vi "Field sweep Generator.vi"(5 "Ramp type":string(combo)="Around origin", 7 "Ramp up first T":bool, 9 "Field Radius":dbl=0.002 format="%#_13g", 10 "Field step":dbl=0.002 format="%#_13g", 11 "Field Origin":dbl=0.002 format="%#_13g") -> (3 "output array":dbl[](array[numeric]))   [LabVIEW 2021]
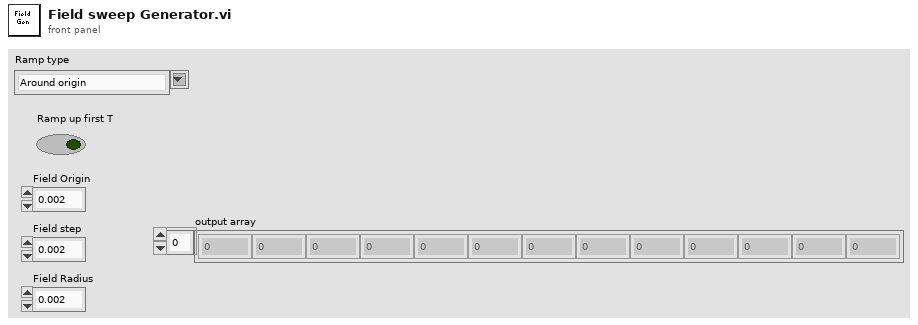
[diagram p1: front panel]
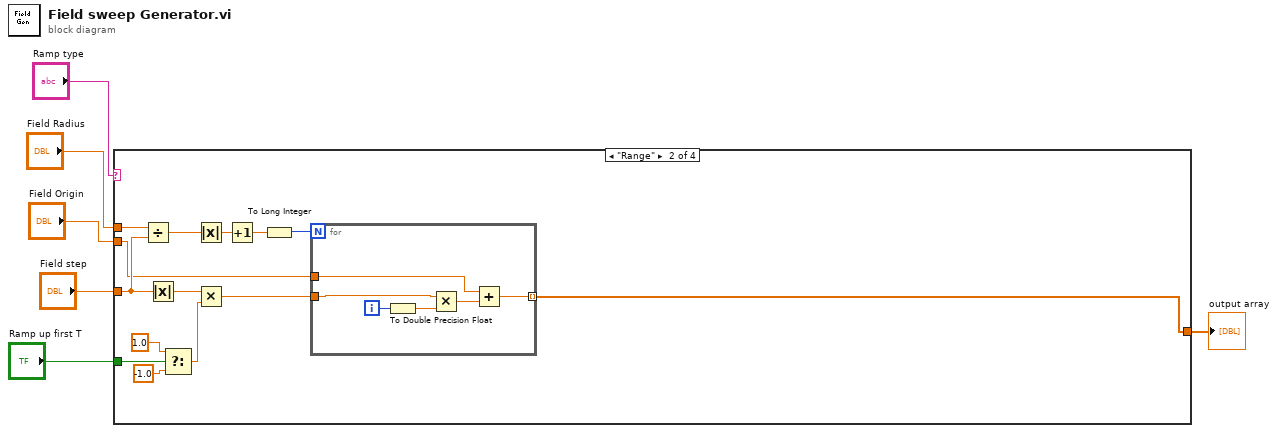
[diagram p0: block diagram]
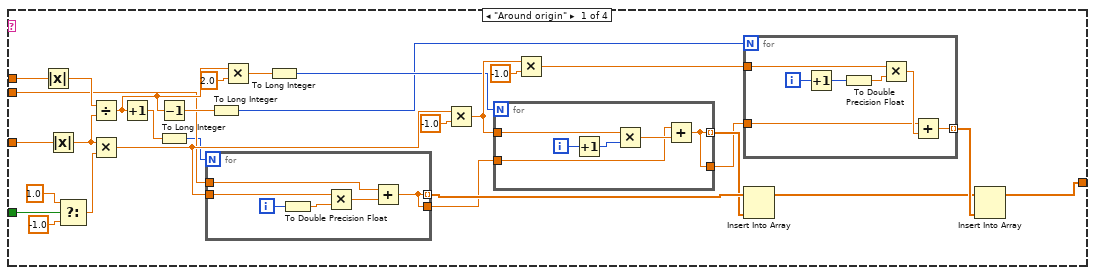
[diagram p2: hidden frame]
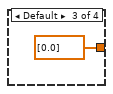
[diagram p3: hidden frame]
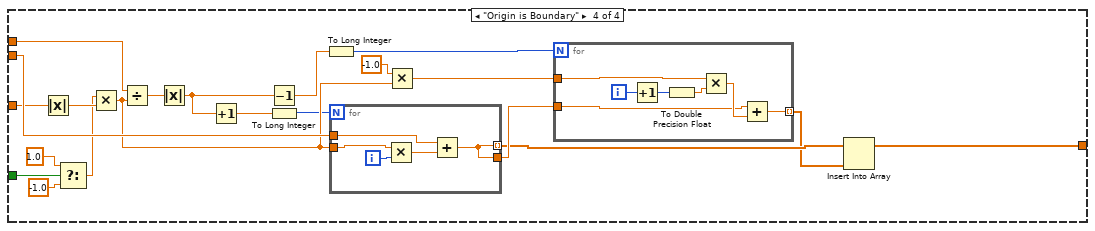
[diagram p4: hidden frame]
diagram:
  n1 = case shown="\"Range\"" "Ramp type" {
    tunnel: [w35 w62 dbl[] [0.0] w84] -> w6
    tunnel: "Ramp up first T" -> [w34 w59 _ w82]
    tunnel: "Field Radius" -> [w31 w68 _ w96]
    tunnel: "Field step" -> [w25 w64 _ w90]
    tunnel: "Field Origin" -> [w10 w63 _ w93]
    frame "Around origin" {
      n2 = Absolute Value(x=w31) -> (abs(x)=w30:dbl)
      n3 = Absolute Value(x=w25) -> (abs(x)=w13:dbl)
      n4 = Select(t=1.0, s=w34, f=-1.0) -> (s? t:f=w11:dbl)
      n5 = Divide(x=w30, y=w13) -> (x/y=w18:dbl)
      n6 = Multiply(x=w13, y=w11) -> (x*y=w12:dbl)
      n7 = Increment(x=w18) -> (x+1=w15:dbl)
      n8 = Decrement(x=w18) -> (x-1=w14:dbl)
      n9 = To Long Integer(number=w15) -> (32bit integer=w9:i32)
      n10 = for {
        N: w9 -> [_]
        tunnel: w12 -> [w53]
        tunnel: [w51] -> w29 mode=indexing
        tunnel: [w51] -> w28
        tunnel: w10 -> [w50]
        i -> [w54]
        n11 = To Double Precision Float(number=w54) -> (double precision float=w49:dbl)
        n12 = Multiply(x=w53, y=w49) -> (x*y=w52:dbl)
        n13 = Add(x=w50, y=w52) -> (x+y=w51:dbl)
      }
      n14 = To Long Integer(number=w14) -> (32bit integer=w7:i32)
      n15 = Multiply(x=w18, y=2.0) -> (x*y=w26:dbl)
      n16 = To Long Integer(number=w26) -> (32bit integer=w8:i32)
      n17 = Multiply(x=w12, y=-1.0) -> (x*y=w21:dbl)
      n18 = for {
        N: w8 -> [_]
        tunnel: w21 -> [w47]
        tunnel: w28 -> [w45]
        tunnel: [w43] -> w23 mode=indexing
        tunnel: [w43] -> w22
        i -> [w48]
        n19 = Increment(x=w48) -> (x+1=w44:i32)
        n20 = Multiply(x=w47, y=w44) -> (x*y=w46:dbl)
        n21 = Add(x=w45, y=w46) -> (x+y=w43:dbl)
      }
      n22 = Multiply(x=w21, y=-1.0) -> (x*y=w20:dbl)
      n23 = for {
        N: w7 -> [_]
        tunnel: w20 -> [w41]
        tunnel: w22 -> [w39]
        tunnel: [w38] -> w17 mode=indexing
        i -> [w42]
        n24 = Increment(x=w42) -> (x+1=w37:i32)
        n25 = To Double Precision Float(number=w37) -> (double precision float=w36:dbl)
        n26 = Multiply(x=w41, y=w36) -> (x*y=w40:dbl)
        n27 = Add(x=w39, y=w40) -> (x+y=w38:dbl)
      }
      n28 = Insert Into Array(array=w29, new element=w23) -> (w16:dbl[])  [unwired: 1 in]
      n29 = Insert Into Array(array=w16, new element=w17) -> (w35:dbl[])  [unwired: 1 in]
    }
    frame "Range" {
      n30 = Divide(x=w68, y=w64) -> (x/y=w67:dbl)
      n31 = Absolute Value(x=w64) -> (abs(x)=w60:dbl)
      n32 = Select(t=1.0, s=w59, f=-1.0) -> (s? t:f=w55:dbl)
      n33 = Absolute Value(x=w67) -> (abs(x)=w66:dbl)
      n34 = Multiply(x=w60, y=w55) -> (x*y=w56:dbl)
      n35 = Increment(x=w66) -> (x+1=w65:dbl)
      n36 = To Long Integer(number=w65) -> (32bit integer=w61:i32)
      n37 = for {
        N: w61 -> [_]
        tunnel: w56 -> [w73]
        tunnel: w63 -> [w71]
        tunnel: [w70] -> w62 mode=indexing
        i -> [w74]
        n38 = To Double Precision Float(number=w74) -> (double precision float=w69:dbl)
        n39 = Multiply(x=w73, y=w69) -> (x*y=w72:dbl)
        n40 = Add(x=w71, y=w72) -> (x+y=w70:dbl)
      }
    }
    frame Default {
    }
    frame "Origin is Boundary" {
      n41 = Absolute Value(x=w90) -> (abs(x)=w83:dbl)
      n42 = Select(t=1.0, s=w82, f=-1.0) -> (s? t:f=w78:dbl)
      n43 = Multiply(x=w78, y=w83) -> (x*y=w79:dbl)
      n44 = Divide(x=w96, y=w79) -> (x/y=w95:dbl)
      n45 = Absolute Value(x=w95) -> (abs(x)=w92:dbl)
      n46 = Increment(x=w92) -> (x+1=w94:dbl)
      n47 = Decrement(x=w92) -> (x-1=w91:dbl)
      n48 = To Long Integer(number=w94) -> (32bit integer=w77:i32)
      n49 = To Long Integer(number=w91) -> (32bit integer=w76:i32)
      n50 = for {
        N: w77 -> [_]
        tunnel: w79 -> [w107]
        tunnel: w93 -> [w105]
        tunnel: [w104] -> w86 mode=indexing
        tunnel: [w104] -> w87
        i -> [w108]
        n51 = Multiply(x=w107, y=w108) -> (x*y=w106:dbl)
        n52 = Add(x=w105, y=w106) -> (x+y=w104:dbl)
      }
      n53 = Multiply(x=-1.0, y=w79) -> (x*y=w89:dbl)
      n54 = for {
        N: w76 -> [_]
        tunnel: w89 -> [w101]
        tunnel: w87 -> [w100]
        tunnel: [w98] -> w85 mode=indexing
        i -> [w102]
        n55 = Increment(x=w102) -> (x+1=w99:i32)
        n56 = To Double Precision Float(number=w99) -> (double precision float=w97:dbl)
        n57 = Multiply(x=w101, y=w97) -> (x*y=w103:dbl)
        n58 = Add(x=w100, y=w103) -> (x+y=w98:dbl)
      }
      n59 = Insert Into Array(array=w86, new element=w85) -> (w84:dbl[])  [unwired: 1 in]
    }
  }
  "output array" <- w6
